vi "Parse Search Query.vi"(8 "error in (no error)":errorcluster, 11 "input string":string) -> (0 "error out":errorcluster, 2 "searched objects":string[](array[string]), 3 "search query":T1)   [LabVIEW 2017]
uses:
  Search Query Type.ctl
  <vilib>/regexp/Match Regular Expression.xnode
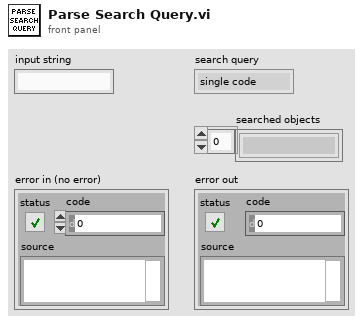
[diagram p1: front panel]
types:
  T1 = typedef "Search Query Type.ctl" = enum16{"single code", "code range", "keywords", "error"}
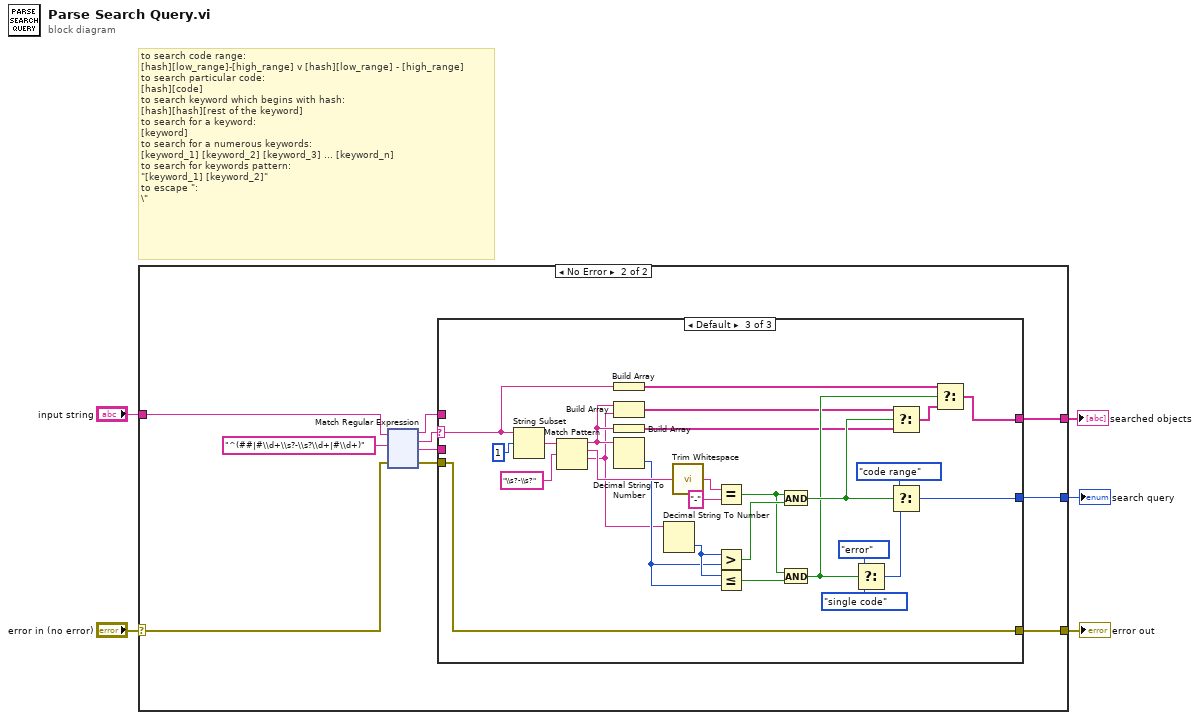
[diagram p0: block diagram]
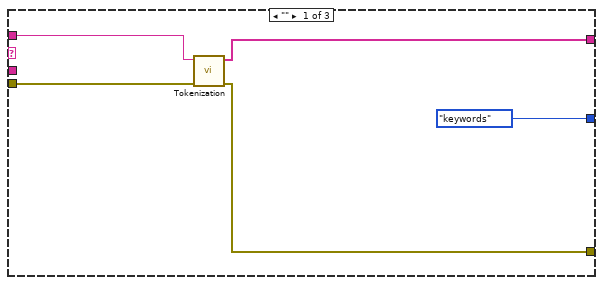
[diagram p3: hidden frame]
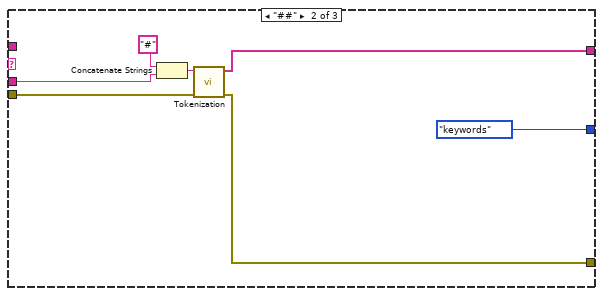
[diagram p4: hidden frame]
diagram:
  # "to search code range:\n[hash][low_range]-[high_range] v [hash][low_range] - [high_range]\nto search particular code:\n[hash][code]\nto search keyword which begins with hash:\n[hash][hash][rest of the keyword]\nto search for a keyword:\n[keyword]\nto search for a numerous keywords:\n[keyword_1] [keyword_2] [keyword_3] ... [keyword_n]\nto search for keywords pattern:\n\"[keyword_1] [keyword_2]\"\nto escape \":\n\\\""
  n1 = case shown="No Error" "error in (no error)" {
    selector: "error in (no error)" -> [w6 w7]
    tunnel: "input string" -> [_ w15]
    tunnel: [_ w11] -> w4
    tunnel: [_ w10] -> w1
    tunnel: [w6 w8] -> w2
    frame Error {
    }
    frame No Error {
      n2 = xnode "Match Regular Expression"("input string"=w15, "regular expression"="^(##|#\\d+\\s?-\\s?\\d+|#\\d+)", "error in"=w7) -> ("before match"=w12:string, "whole match"=w14:string, "after match"=w13:string, "error out"=w9:errorcluster)  [unwired: 3 in, 1 out]
      n3 = case shown="Default" w14 {
        selector: w14 -> [_ _ w35]
        tunnel: w13 -> [_ w28 _]
        tunnel: w12 -> [w21 _ _]
        tunnel: [Search_Query_Type."keywords" Search_Query_Type."keywords" w49] -> w11
        tunnel: [w20 w25 w36] -> w10
        tunnel: w9 -> [w19 w24 w46]
        tunnel: [w18 w23 w46] -> w8
        frame "" {
          n4 = call "Tokenization.vi"("error in (no error)"=w19, "string"=w21) -> ("error out"=w18:errorcluster, "tokens"=w20:string[])  [unwired: 8 in]
        }
        frame "##" {
          n5 = Concatenate Strings("#" ("string"), w28) -> (w26:string)
          n6 = call "Tokenization.vi"("error in (no error)"=w24, "string"=w26) -> ("error out"=w23:errorcluster, "tokens"=w25:string[])  [unwired: 8 in]
        }
        frame Default {
          n7 = String Subset(string=w35, offset (0)=1) -> (substring=w51:string)  [unwired: 1 in]
          n8 = Match Pattern(string=w51, regular expression="\\s?-\\s?") -> (before substring=w33:string, match substring=w54:string, after substring=w32:string)  [unwired: 1 in, 1 out]
          n9 = Build Array(w35) -> (w29:string[])
          n10 = Build Array(w33, w32) -> (w31:string[])
          n11 = Build Array(w33) -> (w30:string[])
          n12 = Decimal String To Number(string=w33) -> (number=w40:i32)  [unwired: 2 in, 1 out]
          n13 = Decimal String To Number(string=w32) -> (number=w41:i32)  [unwired: 2 in, 1 out]
          n14 = call <vilib>:"Trim Whitespace.vi"("string"=w54) -> ("trimmed string"=w53:string)  [unwired: 1 in]
          n15 = Equal?(x=w53, y="-") -> (x = y?=w39:bool)
          n16 = Greater?(x=w41, y=w40) -> (0:w42:bool)
          n17 = Less Or Equal?(x=w41, y=w40) -> (x <= y?=w38:bool)
          n18 = And(x=w39, y=w42) -> (x .and. y?=w47:bool)
          n19 = And(x=w39, y=w38) -> (x .and. y?=w34:bool)
          n20 = Select(t=Search_Query_Type."error", s=w34, f=Search_Query_Type."single code") -> (s? t:f=w43:T1)
          n21 = Select(t=w31, s=w47, f=w30) -> (s? t:f=w37:string[])
          n22 = Select(t=Search_Query_Type."code range", s=w47, f=w43) -> (s? t:f=w49:T1)
          n23 = Select(t=w29, s=w34, f=w37) -> (s? t:f=w36:string[])
        }
      }
    }
  }
  "search query" <- w4
  "error out" <- w2
  "searched objects" <- w1
